vi "CAENHV Get Sys Prop Numeric.vi"(8 "error in (no error)":errorcluster, 10 "PropName":string, 11 "handle":i32) -> (0 "error out":errorcluster, 3 "Result":i16)   [LabVIEW 2009, in "CAENHVWrapper.lvlib"]
doc: "CAENHVLIB_API CAENHVRESULT CAENHV_GetSysProp(int handle, \n const char *PropName, void *Result);"
uses:
  <userlib>/CAENHVWrapper/CAENHVWrapper.lvlib
  <userlib>/CAENHVWrapper/CAENHVWrapper.dll
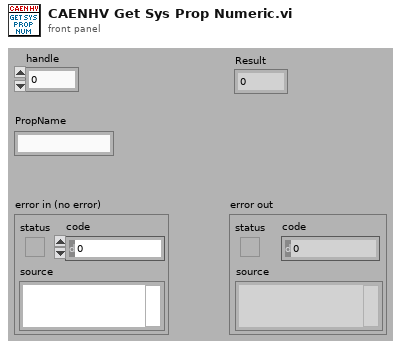
[diagram p1: front panel]
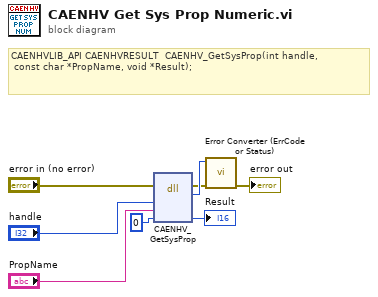
[diagram p0: block diagram]
diagram:
  # "CAENHVLIB_API CAENHVRESULT  CAENHV_GetSysProp(int handle, \n const char *PropName, void *Result);"
  n1 = dll-call lib="C:/Program Files/National Instruments/LabVIEW 2009/user.lib/CAENHVWrapper/CAENHVWrapper.*" fn="CAENHV_GetSysProp"(error in="error in (no error)", "handle"="handle", "PropName"="PropName", "Result"=i16 0) -> (error out=w3:errorcluster, "return type"=w8:i32, "Result"=→"Result":i16)  [unwired: 4 in, 1 out]
  n2 = call <userlib>:"Error Converter (ErrCode or Status).vi"("error in (no error)"=w3, "error code"=w8) -> ("error out"=→"error out":errorcluster)  [unwired: 9 in]
